vi "UART Close.vi"(8 "Error In":errorcluster, 10 "UART Channel (0)":u8, 11 "LINX Resource":T1) -> (0 "Error Out":errorcluster, 3 "LINX Resource":T1)   [LabVIEW 2013, in "LVH-LINX.lvlib"]
doc: "Close the specified UART channel."
uses:
  <vilib>/LabVIEW Hacker/LINX/LVH-LINX.lvlib
  <vilib>/LabVIEW Hacker/LINX/Private/Type Defs/LINX Ref.ctl
  <vilib>/LabVIEW Hacker/LINX/Private/Type Defs/Platform.ctl
  <vilib>/LabVIEW Hacker/LINX/Private/Type Defs/Interface.ctl
  <vilib>/LabVIEW Hacker/LINX/Private/Device/Type Defs/LINX Device Config.ctl
  <vilib>/LabVIEW Hacker/LINX/Private/Device/Type Defs/TCP Config.ctl
  <vilib>/LabVIEW Hacker/LINX/Private/Type Defs/Device Family.ctl
  <vilib>/LabVIEW Hacker/LINX/Private/Type Defs/Peripheral.ctl
  <vilib>/LabVIEW Hacker/LINX/Private/Type Defs/Channel FGV States.ctl
  <vilib>/LabVIEW Hacker/LINX/Private/Device/Device.lvlib
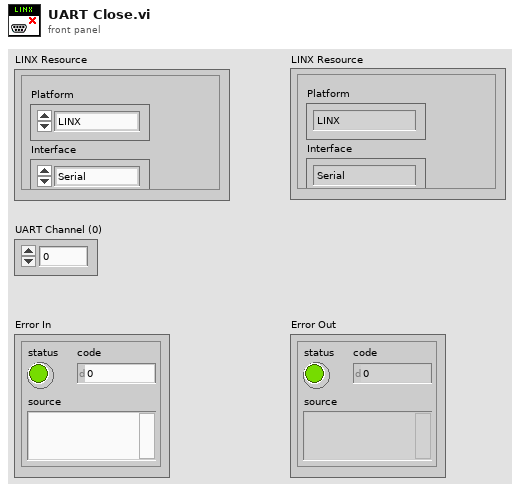
[diagram p1: front panel]
types:
  T1 = typedef "LVH-LINX.lvlib/LINX Ref.ctl" = cluster{"Platform":T2, "Interface":T3, "LINX Device Config":T4}
  T2 = typedef "LVH-LINX.lvlib/Platform.ctl" = enum16{"LINX", "myRIO"}
  T3 = typedef "LVH-LINX.lvlib/Interface.ctl" = enum16{"Serial", "TCP"}
  T4 = typedef "LVH-LINX.lvlib/Device.lvlib/LINX Device Config.ctl" = cluster{"Interface":T3, "COM Port":refnum<visa-resource-name>, "TCP Configuration":T5, "Device Family":T6, "Device ID":u8, "Device Name":string, "TCP Ref":refnum<k5>}
  T5 = typedef "LVH-LINX.lvlib/Device.lvlib/TCP Config.ctl" = cluster{"IP Address":string, "Port":u16}
  T6 = typedef "LVH-LINX.lvlib/Device Family.ctl" = enum8{"National Instruments", "Digilent", "Arduino"}
  T7 = typedef "LVH-LINX.lvlib/Peripheral.ctl" = enum8{"DI", "DO", "AI", "AO", "PWM", "QE", "UART", "I2C", "SPI", "CAN"}
  T8 = typedef "LVH-LINX.lvlib/Channel FGV States.ctl" = enum16{"Initialize", "Get", "Set"}
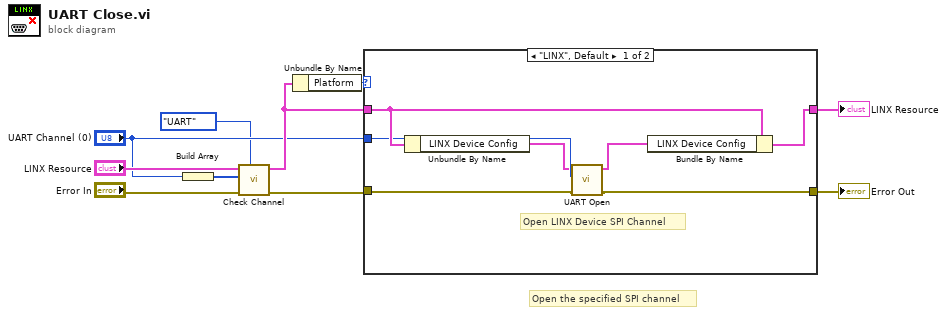
[diagram p0: block diagram]
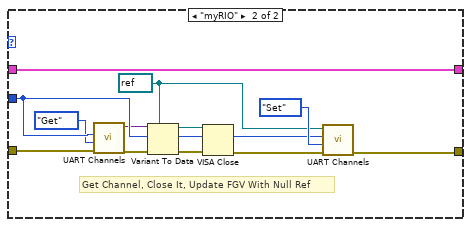
[diagram p2: hidden frame]
diagram:
  # "Open the specified SPI channel"
  n1 = Build Array("UART Channel (0)") -> (w3:u8[])
  n2 = call <vilib>:"Check Channel.vi"("Peripheral"=Peripheral."UART", "Error In"="Error In", "Channels"=w3, "LINX Resource"="LINX Resource") -> ("Error Out"=w4:errorcluster, "LINX Resource"=w5:T1)  [unwired: 5 in, 1 out]
  n3 = Unbundle By Name(w5) -> ("Platform"=w10:T2)
  n4 = case shown="\"LINX\", Default" w10 {
    tunnel: w4 -> [w14 w26]
    tunnel: w5 -> [w17 w29]
    tunnel: [w15 w27] -> w9
    tunnel: [w16 w29] -> w8
    tunnel: "UART Channel (0)" -> [w13 w25]
    frame "LINX", Default {
      # "Open LINX Device SPI Channel"
      n5 = Unbundle By Name(w17) -> ("LINX Device Config"=w12:T4)
      n6 = call <vilib>:"UART Open.vi"("Error In"=w14, "UART Channel"=w13, "LINX Device Config"=w12) -> ("Error Out"=w15:errorcluster, "LINX Device Config"=w11:T4)  [unwired: 7 in]
      n7 = Bundle By Name(cluster=w17, "LINX Device Config"=w11) -> (w16:T1)
    }
    frame "myRIO" {
      w18 = refnum<visa-resource-name> refnum ("VISA resource name")
      # "Get Channel, Close It, Update FGV With Null Ref"
      n8 = call <vilib>:"UART Channels.vi"("Error In"=w26, "Channel State"=Channel_FGV_States."Get", "Channel Number"=w25) -> ("Error Out"=w22:errorcluster, "UART Channel"=w21:variant)  [unwired: 7 in]
      n9 = Variant To Data(error in=w22, type=w18, Variant=w21) -> (data=w20:refnum<visa-resource-name>, error out=w23:errorcluster)
      n10 = VISA Close(VISA resource name=w20, error in (no error)=w23) -> (error out=w19:errorcluster)
      n11 = call <vilib>:"UART Channels.vi"("Error In"=w19, "Channel State"=Channel_FGV_States."Set", "Channel Number"=w25, "UART Channel"=w18) -> ("Error Out"=w27:errorcluster)  [unwired: 6 in, 1 out]
    }
  }
  "Error Out" <- w9
  "LINX Resource" <- w8
